vi "ParseAMIResponce.vi"(11 "Responce":u8[](array[numeric])=[2, 48, 49, 65, 77, 73, 44, 79, 75, 44, 84, 69, 77, 80, 45, 50, 48, 48, 48, 32, 32, 86, 48, 48, 45, 82, 48, 48, 50, 52, 13, 10] format="%x") -> (1 "Version-Revision":u8[](array[numeric]), 2 "Model Name":u8[](array[numeric]), 3 "Result Code":i8)   [LabVIEW 2015]
uses:
  <instrlib>/Samwontech TEMP2xxx/Samwontech TEMP2xxx.lvlib
panel:
  out "Version-Revision":string
  out "Model Name":string
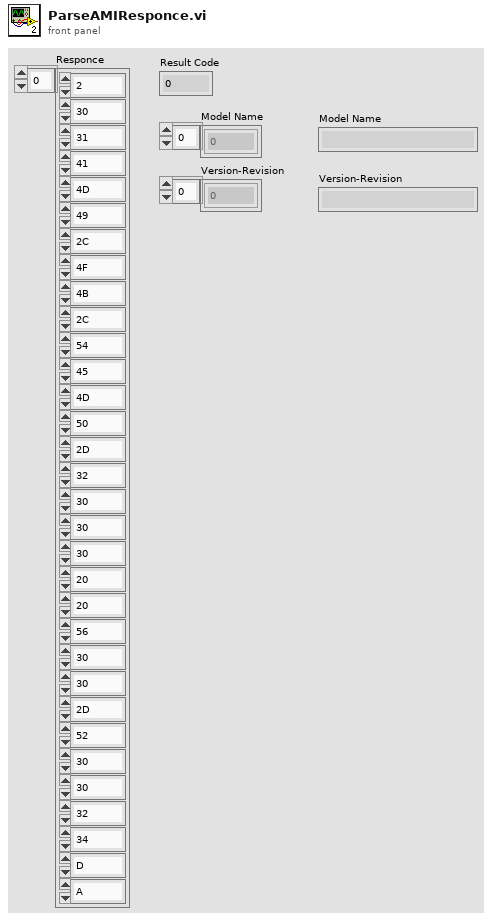
[diagram p1: front panel]
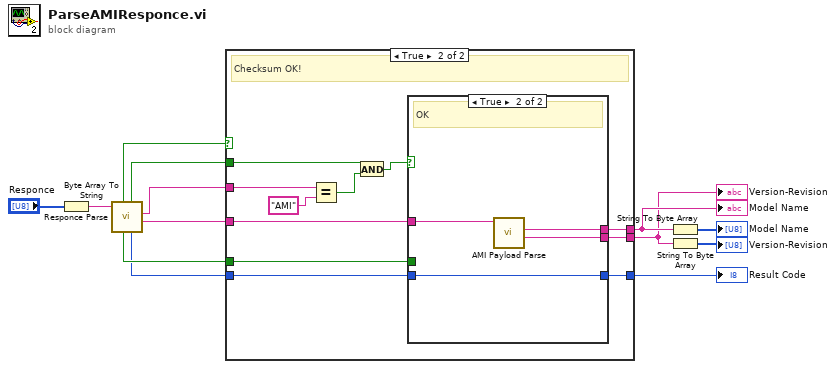
[diagram p0: block diagram]
diagram:
  n1 = Byte Array To String(unsigned byte array="Responce") -> (string=w6:string)
  n2 = call <instrlib>:"Responce Parse.vi"("Responce"=w6) -> ("Payload"=w9:string, "Command"=w1:string, "Error Code"=w11:i8, "OK"=w10:bool, "Error?"=w12:bool, "Checksum OK"=w13:bool)  [unwired: 4 in, 1 out]
  n3 = case shown="True" w13 {
    tunnel: w12 -> [_ w21]
    tunnel: w11 -> [_ w20]
    tunnel: w10 -> [_ w15]
    tunnel: w9 -> [_ w24]
    tunnel: [_ w23] -> w5
    tunnel: [_ w22] -> w4
    tunnel: [_ w19] -> w8
    tunnel: w1 -> [_ w17]
    frame False {
    }
    frame True {
      # "Checksum OK!"
      n4 = Equal?(x=w17, y="AMI") -> (x = y?=w14:bool)
      n5 = And(x=w15, y=w14) -> (x .and. y?=w16:bool)
      n6 = case shown="True" w16 {
        tunnel: w24 -> [_ w29]
        tunnel: [_ w28] -> w23
        tunnel: [_ w27] -> w22
        tunnel: w21 -> [_ _]
        tunnel: w20 -> [w25 w26]
        tunnel: [w25 w26] -> w19
        frame False {
          # "Not OK"
        }
        frame True {
          # "OK"
          n7 = call <instrlib>:"AMI Payload Parse.vi"("Payload"=w29) -> ("Version-Revision"=w27:string, "Model Name"=w28:string)  [unwired: 8 in, 1 out]
        }
      }
    }
  }
  "Result Code" <- w8
  "Model Name" <- w5
  "Version-Revision" <- w4
  n8 = String To Byte Array(string=w5) -> (unsigned byte array=→"Model Name":u8[])
  n9 = String To Byte Array(string=w4) -> (unsigned byte array=→"Version-Revision":u8[])
